vi "ImplementInterfaces.vi"(0 "ClassWriterNative":refnum<class "ClassWriterNative.lvclass">, 1 "ClassItemRefIn":refnum<vi>, 2 "InterfacesToImplement":T1, 5 "error in (no error)":errorcluster) -> (14 "ClassWriterNative":refnum<class "ClassWriterNative.lvclass">, 15 "ClassItemRefOut":refnum<vi>, 17 "Cancelled":bool, 19 "error out":errorcluster)   [LabVIEW 2020, in "ClassWriterNative.lvclass"]
uses:
  <resource>/Framework/Providers/Open_GDS/ClassProviders/Provider_LvNativeClass/ClassWriterNative_class/ClassWriterNative.lvclass
  C:/Program Files (x86)/National Instruments/LabVIEW 2020/resource/Framework/Providers/Open_GDS/ClassProviders/Provider_BaseClassInterface/ClassWriter_class/ClassWriter.lvclass
  <resource>/Framework/Providers/Open_GDS/ClassProviders/Provider_BaseClassInterface/ClassWriter_class/InterfacesToImplement.ctl
  <resource>/Framework/Providers/Open_GDS/ClassProviders/Common/InterfaceLibrary/InterfaceLibrary.lvlib
  <resource>/Framework/Providers/Open_GDS/ClassProviders/Provider_BaseClassInterface/ClassWriter_class/ClassWriter.lvclass
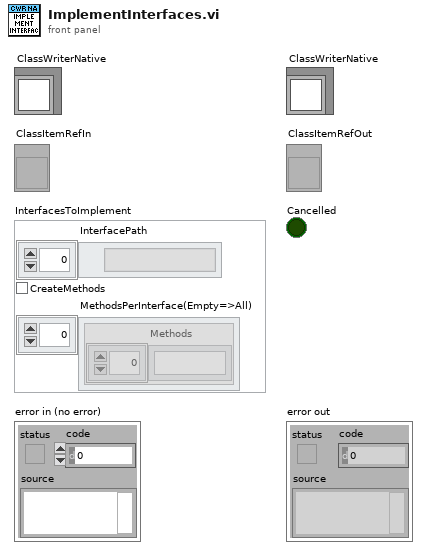
[diagram p1: front panel]
types:
  T1 = typedef "ClassWriter.lvclass/InterfacesToImplement.ctl" = cluster{"InterfacePath":path[], "CreateMethods":bool, "MethodsPerInterface(Empty=>All)":cluster{"Methods":string[]}[]}
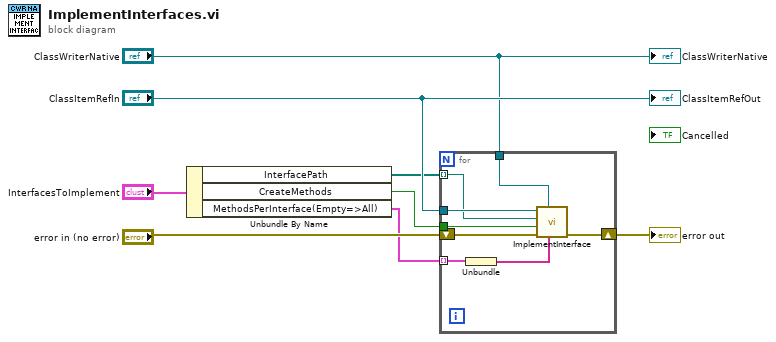
[diagram p0: block diagram]
diagram:
  n1 = Unbundle By Name("InterfacesToImplement") -> ("InterfacePath"=w4:path[], "CreateMethods"=w2:bool, "MethodsPerInterface(Empty=>All)"=w1:cluster{"Methods":string[]}[])
  n2 = for {
    tunnel: "ClassItemRefIn" -> [w14]
    shift-right: [w16] -> w8
    shift-left: "error in (no error)" -> [w15]
    tunnel: w4 -> [w13] mode=indexing
    tunnel: "ClassWriterNative" -> [w12]
    tunnel: w2 -> [w11]
    tunnel: w1 -> [w10] mode=indexing
    n3 = Unbundle(w10) -> ("Methods"=w9:string[])
    n4 = call <resource>:"ImplementInterface.vi"("InterfaceMethodsToCreate"=w9, "ClassWriter.lvclass"=w12, "error in"=w15, "CreateMethods"=w11, "Interface Path"=w13, "LvClassPath/LvClassProjectItem"=w14) -> ("error out"=w16:errorcluster)  [unwired: 5 in]
  }
  "error out" <- w8
  "ClassWriterNative" <- "ClassWriterNative"
  "ClassItemRefOut" <- "ClassItemRefIn"
